vi "TMaitai.vi"() -> ()   [LabVIEW 2011]
panel:
  in  "timeout in ms (for status check)":i32=3000
  out "end?":bool
  in  "error in (no error)":errorcluster
  out "value out":string
  out "error out":errorcluster
  out "value":string
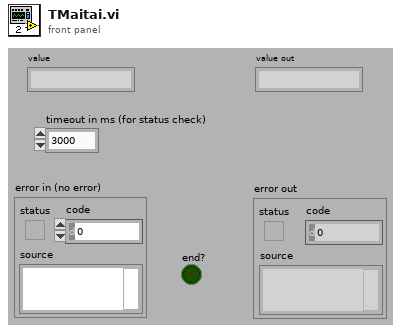
[diagram p1: front panel]
types:
  T1 = cluster{"command":string, "variable":string, "return":string}[]
  T2 = enum16{"None/#Datasets", "Clear", "TagValueOf#", "AddValues", "ReadValue", "ChangeValue", "Get all"}
  T3 = cluster{"command":string, "variable":string, "return":string}
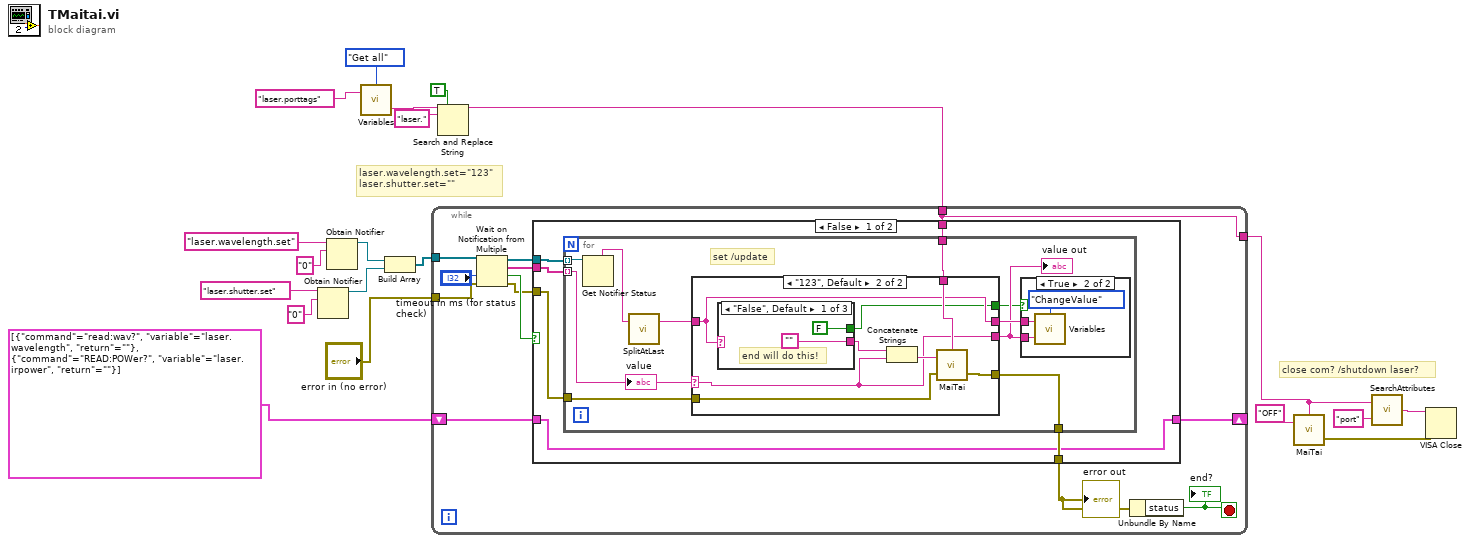
[diagram p0: block diagram]
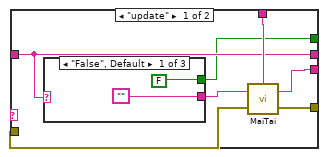
[diagram p3: hidden frame]
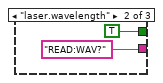
[diagram p4: hidden frame]
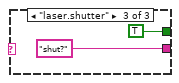
[diagram p5: hidden frame]
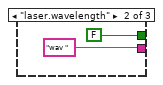
[diagram p6: hidden frame]
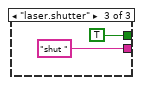
[diagram p7: hidden frame]
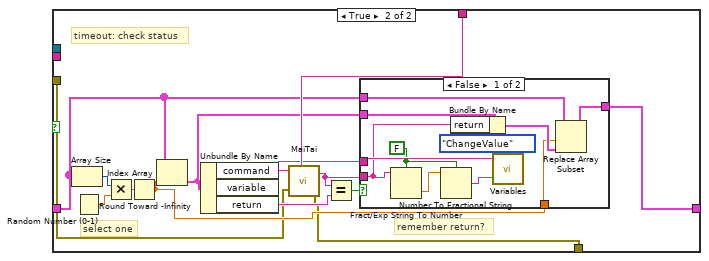
[diagram p8: hidden frame]
diagram:
  # "close com? /shutdown laser?"
  # "laser.wavelength.set=\"123\"\nlaser.shutter.set=\"\""
  n1 = Obtain Notifier(name (unnamed)="laser.shutter.set", notification data type="0") -> (notifier out=w6:refnum<notifier>)  [unwired: 2 in, 2 out]
  n2 = Obtain Notifier(name (unnamed)="laser.wavelength.set", notification data type="0") -> (notifier out=w13:refnum<notifier>)  [unwired: 2 in, 2 out]
  n3 = call "Variables.vi"("Tag in"="laser.porttags", "Command"=T2."Get all") -> ("value out"=w17:string)  [unwired: 1 in, 2 out]
  n4 = Build Array(w13, w6) -> (w7:refnum<notifier>[])
  n5 = Search and Replace String(replace all?=TRUE ("replace all? (F)"), input string=w17, search string="laser.") -> (result string=w11:string)  [unwired: 1 in, 7 out]
  n6 = while {
    tunnel: "error in (no error)" -> [w24]
    tunnel: w11 -> [w23]
    tunnel: w7 -> [w32]
    shift-right: [w27] -> _
    shift-left: T1 [{"command"="read:wav?", "variable"="laser.wavelength", "return"=""}, {"command"="READ:POWer?", "variable"="laser.irpower", "return"=""}] -> [w28]
    tunnel: [w23] -> w3
    stop <- w31 stop-if-true
    n7 = Wait on Notification from Multiple(0:w32, 2:"timeout in ms (for status check)", 3:w24) -> (8:w25:refnum<notifier>[], 9:w30:string[], 10:w29:bool, 11:w22:errorcluster)  [unwired: 1 out]
    n8 = case shown="False" w29 {
      tunnel: w30 -> [w38 _]
      tunnel: w22 -> [w37 w80]
      tunnel: w23 -> [w36 w93]
      tunnel: [w35 w79] -> w21
      tunnel: w28 -> [w34 w83]
      tunnel: [w34 w82] -> w27
      tunnel: w25 -> [w33 _]
      frame False {
        n9 = for {
          tunnel: w38 -> [w40] mode=indexing
          tunnel: w37 -> [w47]
          tunnel: w36 -> [w46]
          tunnel: [w45] -> w35
          tunnel: w33 -> [w42] mode=indexing
          # "set /update"
          n10 = Get Notifier Status(notifier=w42) -> (notifier name=w41:string)  [unwired: 1 in, 4 out]
          n11 = call "SplitAtLast.vi"("In-String"=w41) -> ("Front (default)"=w48:string)  [unwired: 1 in, 1 out]
          n12 = case shown="\"123\", Default" w40 {
            selector: w40 -> [_ w66]
            tunnel: w48 -> [w53 w67]
            tunnel: [w53 w67] -> w44
            tunnel: w47 -> [w56 w71]
            tunnel: w46 -> [w58 w69]
            tunnel: [w55 w68] -> w45
            tunnel: [w54 w66] -> w43
            tunnel: [w52 w65] -> w39
            frame "update" {
              n13 = case shown="\"False\", Default" w53 {
                tunnel: ["" "READ:WAV?" ("string") "shut?" ("string")] -> w57
                tunnel: [FALSE TRUE TRUE] -> w52
                frame "False", Default {
                }
                frame "laser.wavelength" {
                }
                frame "laser.shutter" {
                }
              }
              n14 = call "MaiTai.vi"("error in (no error)"=w56, "command"=w57, "com parameters"=w58) -> ("error out"=w55:errorcluster, "read"=w54:string)  [unwired: 1 out]
            }
            frame "123", Default {
              n15 = case shown="\"False\", Default" w67 {
                tunnel: ["" "wav " ("string") "shut " ("string")] -> w72
                tunnel: [FALSE FALSE TRUE] -> w65
                frame "False", Default {
                  # "end will do this!"
                }
                frame "laser.wavelength" {
                }
                frame "laser.shutter" {
                }
              }
              n16 = Concatenate Strings(w72, w66) -> (w70:string)
              n17 = call "MaiTai.vi"("error in (no error)"=w71, "command"=w70, "com parameters"=w69) -> ("error out"=w68:errorcluster)  [unwired: 2 out]
            }
          }
          "value out" <- w43
          n18 = case shown="True" w39 {
            tunnel: w44 -> [_ w50]
            tunnel: w43 -> [_ w49]
            frame False {
            }
            frame True {
              n19 = call "Variables.vi"("value"=w49, "Tag in"=w50, "Command"=T2."ChangeValue") -> ()  [unwired: 3 out]
            }
          }
          "value" <- w40
        }
      }
      frame True {
        # "remember return?"
        # "select one"
        # "timeout: check status"
        n20 = Array Size(array=w83) -> (size(s)=w92:i32)
        n21 = Random Number (0-1)() -> (number: 0 to 1=w91:dbl)
        n22 = Multiply(x=w92, y=w91) -> (x*y=w90:dbl)
        n23 = Round Toward -Infinity(1:w90) -> (0:w81:dbl)
        n24 = Index Array(array=w83, index=w81) -> (element=w84:T3)
        n25 = Unbundle By Name(w84) -> ("command"=w89:string, "variable"=w88:string, "return"=w85:string)
        n26 = call "MaiTai.vi"("error in (no error)"=w80, "command"=w89, "com parameters"=w93) -> ("error out"=w79:errorcluster, "read"=w87:string)  [unwired: 1 out]
        n27 = Equal?(x=w87, y=w85) -> (x = y?=w86:bool)
        n28 = case shown="False" w86 {
          tunnel: w88 -> [w103 _]
          tunnel: w87 -> [w97 _]
          tunnel: w84 -> [w102 _]
          tunnel: [w99 w105] -> w82
          tunnel: w83 -> [w100 w105]
          tunnel: w81 -> [w98 _]
          frame False {
            w95 = FALSE ("use system decimal point (T)")
            n29 = Fract/Exp String To Number(use system decimal point (T)=w95, string=w97) -> (number=w96:dbl)  [unwired: 3 out]
            n30 = Number To Fractional String(use system decimal point (T)=w95, number=w96) -> (F-format string=w94:string)  [unwired: 2 out]
            n31 = Bundle By Name(cluster=w102, "return"=w97) -> (w101:T3)
            n32 = call "Variables.vi"("value"=w94, "Tag in"=w103, "Command"=T2."ChangeValue") -> ()  [unwired: 3 out]
            n33 = Replace Array Subset(array=w100, new element=w101, index=w98) -> (w99:T1)
          }
          frame True {
          }
        }
      }
    }
    "error out" <- w21
    n34 = Unbundle By Name(w21) -> ("status"=w31:bool)
    "end?" <- w31
  }
  n35 = call "MaiTai.vi"("command"="OFF", "com parameters"=w3) -> ("error out"=w1:errorcluster)  [unwired: 1 in, 2 out]
  n36 = call "SearchAttributes.vi"("Search"="port", "String"=w3) -> ("ValueText"=w5:string)
  n37 = VISA Close(VISA resource name=w5, error in (no error)=w1) -> ()  [unwired: 1 out]
